vi "GenNewTraj.vi"(0 "Points in":cluster{"x":dbl, "y":dbl, "th":dbl}[](array[cluster]), 1 "Turn Rate":dbl=5.0 format="%#_13g", 3 "WaypointsOverride":cluster{"x":dbl, "y":dbl, "th":dbl}[](array[cluster]), 5 "Parameters":T7 {"Limits"."StoopidFast (fps)" min=0.0; "Limits"."Jerk (fps^3)" min=0.0 step=1.0; "Limits"."Accel (fps^2)" min=0.0; "Limits"."Velocity (fps)" min=0.0; "Overrides"."Angle Override" step=5.0; "Overrides"."Velocity Override" step=5.0; "Overrides"."Angular Override" step=5.0; "Angular Limits"."Jerk (deg/s^3)" min=0.0 step=1.0; "Angular Limits"."Accel (deg/s^2)" min=0.0; "Angular Limits"."Velocity (deg/s)" min=0.0}, 7 "Path Type":T8, 9 "TrajTime":dbl format="%#_13g", 11 "Stoopid Overlap %":dbl min=0.0, 12 "Drive Type":T3, 14 "Trajectory Data In Override":T2(array[cluster])) -> (4 "Updated Waypoints":cluster{"x":dbl, "y":dbl, "th":dbl}[](array[cluster]), 6 "Trajectory Data":T2(array[cluster]), 10 "Valid":bool, 15 "Time & Dist":cluster{"Time (s)":dbl, "Distance (ft)":dbl})   [LabVIEW 2025]
uses:
  Types/Path Type.ctl
  Types/Limits.ctl
  Types/Overrides.ctl
  Types/Angluar Limits.ctl
  Types/Drive Type.ctl
  Types/Segment Type.ctl
  Bezier/Bezier Trajectory.vi
  Clothoid/Generate Clothoid Trajectory.vi
panel:
  out "size(s)":i32
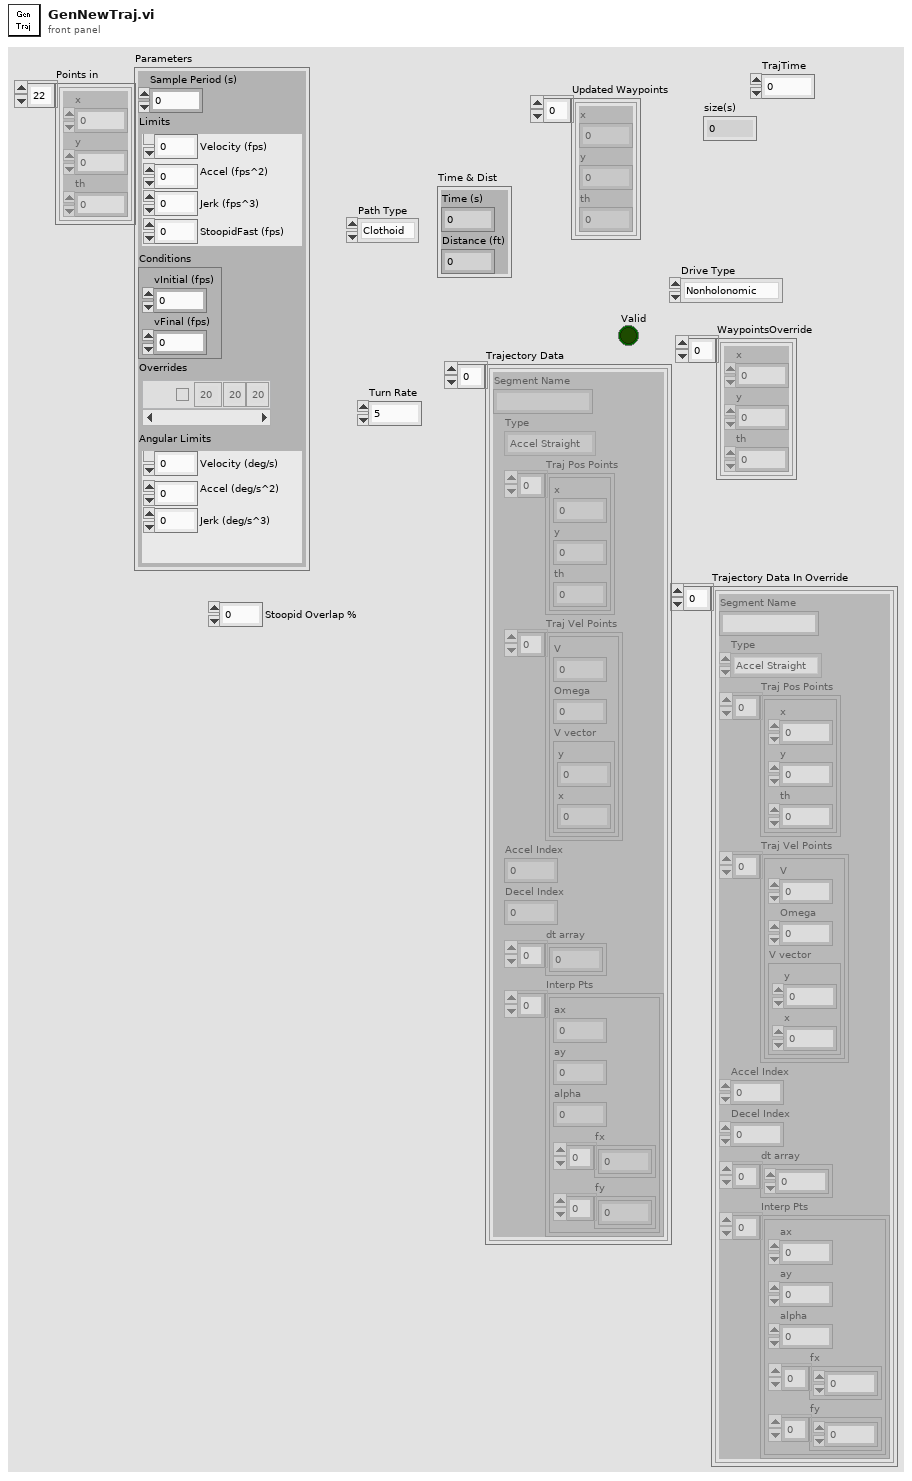
[diagram p1: front panel]
types:
  T1 = typedef "Segment Type.ctl" = enum16{"Accel Straight", "Const Straight", "Blend", "Circle", "Bezier", "Choreo"}
  T2 = cluster{"Segment Name":string, "Type":T1, "Traj Pos Points":cluster{"x":dbl, "y":dbl, "th":dbl}[], "Traj Vel Points":cluster{"V":dbl, "Omega":dbl, "V vector":cluster{"y":dbl, "x":dbl}}[], "Accel Index":i32, "Decel Index":i32, "dt array":dbl[], "Interp Pts":cluster{"ax":dbl, "ay":dbl, "alpha":dbl, "fx":dbl[], "fy":dbl[]}[]}[]
  T3 = typedef "Drive Type.ctl" = enum16{"Nonholonomic", "Holonomic"}
  T4 = typedef "Limits.ctl" = cluster{"Velocity (fps)":dbl, "Accel (fps^2)":dbl, "Jerk (fps^3)":dbl, "StoopidFast (fps)":dbl}
  T5 = typedef "Overrides.ctl" = cluster{"Count":string, "Angular Override":dbl, "Enabled?":bool, "Velocity Override":dbl, "Angle Override":dbl}[]
  T6 = typedef "Angluar Limits.ctl" = cluster{"Velocity (deg/s)":dbl, "Accel (deg/s^2)":dbl, "Jerk (deg/s^3)":dbl}
  T7 = cluster{"Sample Period (s)":dbl, "Limits":T4, "Conditions":cluster{"vInitial (fps)":dbl, "vFinal (fps)":dbl}, "Overrides":T5, "Angular Limits":T6}
  T8 = typedef "Path Type.ctl" = enum16{"Clothoid", "Bezier", "Choreo"}
  T9 = cluster{"vInitial (fps)":dbl, "vFinal (fps)":dbl}
  T10 = cluster{"Segment Name":string, "Type":T1, "Traj Pos Points":cluster{"x":dbl, "y":dbl, "th":dbl}[], "Traj Vel Points":cluster{"V":dbl, "Omega":dbl, "V vector":cluster{"y":dbl, "x":dbl}}[], "Accel Index":i32, "Decel Index":i32, "dt array":dbl[], "Interp Pts":cluster{"ax":dbl, "ay":dbl, "alpha":dbl, "fx":dbl[], "fy":dbl[]}[]}
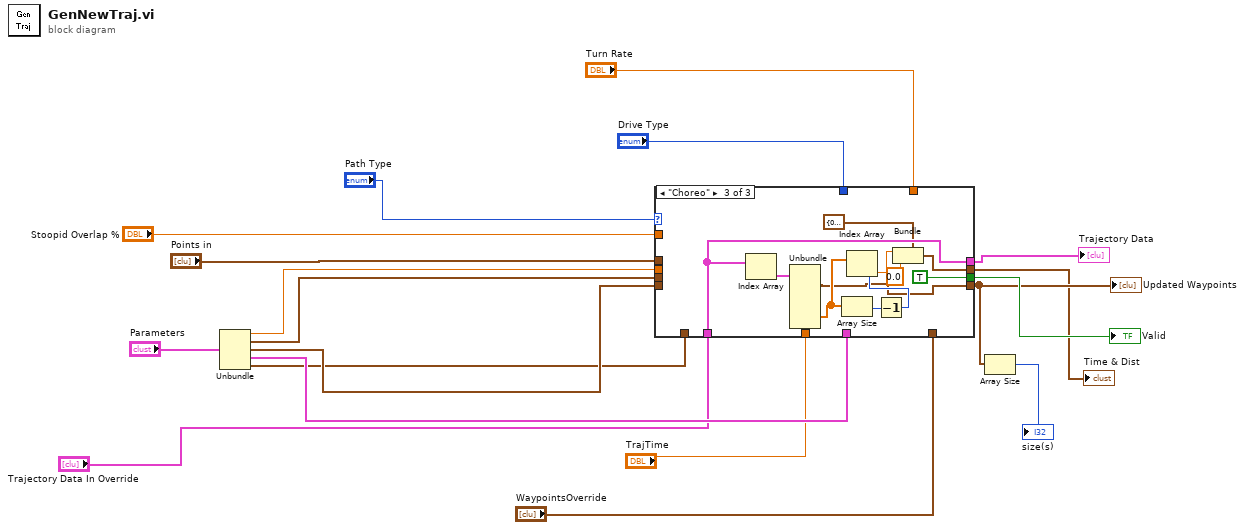
[diagram p0: block diagram]
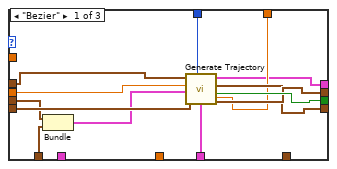
[diagram p2: hidden frame]
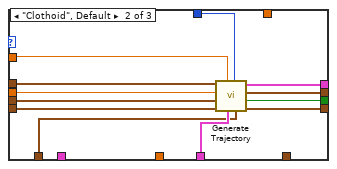
[diagram p3: hidden frame]
diagram:
  n1 = Unbundle("Parameters") -> ("Sample Period (s)"=w13:dbl, "Limits"=w15:T4, "Conditions"=w14:T9, "Overrides"=w17:T5, "Angular Limits"=w11:T6)
  n2 = case shown="\"Choreo\"" "Path Type" {
    tunnel: [w29 w44 TRUE ("Valid")] -> w19
    tunnel: [w28 w43 w47] -> w3
    tunnel: w14 -> [w31 w42 _]
    tunnel: w15 -> [w24 w41 _]
    tunnel: w17 -> [w30 w40 _]
    tunnel: [w27 w39 w45] -> w5
    tunnel: [w20 w33 w54] -> w1
    tunnel: "Stoopid Overlap %" -> [_ w38 _]
    tunnel: "Points in" -> [w32 w37 _]
    tunnel: w13 -> [w26 w36 _]
    tunnel: "Drive Type" -> [w25 w35 _]
    tunnel: w11 -> [w23 w34 _]
    tunnel: "Turn Rate" -> [w21 _ _]
    tunnel: "WaypointsOverride" -> [_ _ _]
    tunnel: "Trajectory Data In Override" -> [_ _ w54]
    tunnel: "TrajTime" -> [_ _ _]
    frame "Bezier" {
      n3 = Bundle("Limits"=w24, "Angular Limits"=w23) -> (w22:cluster{"Limits":T4, "Angular Limits":T6})  [unwired: 1 in]
      n4 = call-poly "Generate Trajectory.vi"("Turn Rate"=w21, "Overrides"=w30, "Drive Type"=w25, "Conditions"=w31, "All Limits"=w22, "sample period (s)"=w26, "WayPoints"=w32) -> ("Time & Dist"=w28:cluster{"Time (s)":dbl, "Distance (ft)":dbl}, "Valid"=w29:bool, "Updated Waypoints"=w27:cluster{"x":dbl, "y":dbl, "th":dbl}[], "Trajectory Data"=w20:T2)  [unwired: 1 in]
    }
    frame "Clothoid", Default {
      n5 = call-poly "Generate Trajectory.vi"("Angular Limits"=w34, "Drive Type"=w35, "Overrides"=w40, "Stoopid Overlap %"=w38, "Conditions"=w42, "Limits"=w41, "Sample Period (s)"=w36, "WayPoints"=w37) -> ("Updated Waypoints"=w39:cluster{"x":dbl, "y":dbl, "th":dbl}[], "Valid"=w44:bool, "Time & Dist"=w43:cluster{"Time (s)":dbl, "Distance (ft)":dbl}, "Traj Data"=w33:T2)
    }
    frame "Choreo" {
      n6 = Index Array(array=w54) -> (element=w53:T10)  [unwired: 1 in]
      n7 = Unbundle(w53) -> ("Traj Pos Points"=w45:cluster{"x":dbl, "y":dbl, "th":dbl}[], "dt array"=w51:dbl[])  [unwired: 6 out]
      n8 = Array Size(array=w51) -> (size(s)=w52:i32)
      n9 = Decrement(x=w52) -> (x-1=w50:i32)
      n10 = Index Array(array=w51, index=w50) -> (element=w49:dbl)
      n11 = Bundle(cluster=cluster{"Time (s)":dbl, "Distance (ft)":dbl} {"Time (s)"=0.0, "Distance (ft)"=0.0} ("Time & Dist"), "Time (s)"=w49, "Distance (ft)"=0.0) -> (w47:cluster{"Time (s)":dbl, "Distance (ft)":dbl})
    }
  }
  "Valid" <- w19
  "Updated Waypoints" <- w5
  "Time & Dist" <- w3
  "Trajectory Data" <- w1
  n12 = Array Size(array=w5) -> (size(s)=→"size(s)":i32)
